vi "3Dmodel.vi"() -> (1 "SceneObject out":refnum<vi>, 2 "error out":errorcluster)   [LabVIEW 2021]
doc: "Creates the 3D scene with the lightsaber composed by two cylinders: the Blade and the Handle."
uses:
  <vilib>/picture/3D Picture Control/Object/Create Object (name).vi
  <vilib>/picture/3D Picture Control/NI_3D Picture Control.lvlib
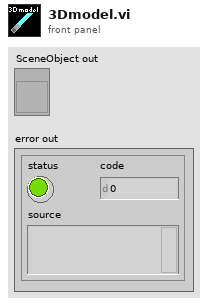
[diagram p1: front panel]
types:
  T1 = cluster{"Red":sgl, "Green":sgl, "Blue":sgl, "Alpha":sgl}
  T2 = enum16{"As a Decal", "With Modulation", "With Blending", "As a replacement"}
  T3 = typedef "imagedata.ctl" = cluster{"image type":i32, "image depth":i32, "image":u8[], "mask":u8[], "colors":u32[], "Rectangle":cluster{"left":i16, "top":i16, "right":i16, "bottom":i16}}
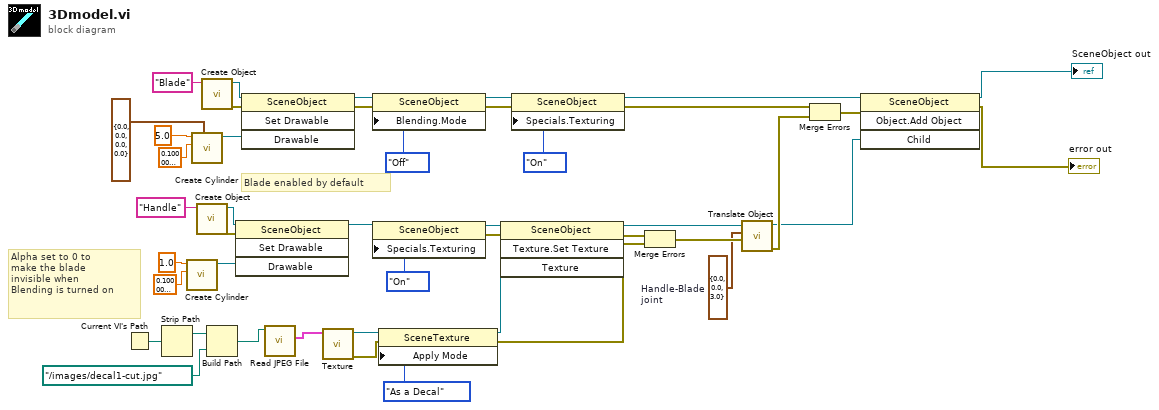
[diagram p0: block diagram]
diagram:
  w23 = cluster{"X":sgl, "Y":sgl, "Z":sgl} {"X"=0.0, "Y"=0.0, "Z"=3.0}  # Handle-Blade joint
  # "Blade enabled by default"
  # "Alpha set to 0 to \nmake the blade\ninvisible when \nBlending is turned on"
  n1 = Current VI's Path() -> (path=w5:path)
  n2 = Strip Path(path=w5) -> (stripped path=w6:path)  [unwired: 1 out]
  n3 = call <vilib>:"Create Cylinder.vi"("Radius"=sgl 0.1, "Height"=sgl 1.0) -> ("New Cylinder Refnum"=w22:refnum<vi>)  [unwired: 8 in, 1 out]
  n4 = call <vilib>:"Create Cylinder.vi"("Color"=T1 {"Red"=0.0, "Green"=0.0, "Blue"=0.0, "Alpha"=0.0}, "Radius"=sgl 0.1, "Height"=sgl 5.0) -> ("New Cylinder Refnum"=w19:refnum<vi>)  [unwired: 7 in, 1 out]
  n5 = call-poly <vilib>:"Create Object.vi"("Name"="Handle") -> ("error out"=w28:errorcluster, "Scene:New Object"=w25:refnum<vi>)  [unwired: 9 in]
  n6 = call-poly <vilib>:"Create Object.vi"("Name"="Blade") -> ("error out"=w14:errorcluster, "Scene:New Object"=w15:refnum<vi>)  [unwired: 9 in]
  n7 = Build Path(base path=w6, name or relative path=path "../images/decal1-cut.jpg" ("path to JPEG file")) -> (appended path=w3:path)
  n8 = invoke class="SceneObject" method="Set Drawable"(reference=w25, error in=w28, "Drawable"=w22) -> (reference out=w41:refnum<vi>)  [unwired: 1 in, 3 out]
  n9 = invoke class="SceneObject" method="Set Drawable"(reference=w15, error in=w14, "Drawable"=w19) -> (reference out=w13:refnum<vi>, error out=w12:errorcluster)  [unwired: 1 in, 2 out]
  n10 = call <vilib>:"Read JPEG File.vi"("path to JPEG file"=w3) -> ("image data"=w34:T3)  [unwired: 8 in, 2 out]
  n11 = call <vilib>:"Texture.vi"("Image"=w34) -> ("error out"=w36:errorcluster, "New Texture Refnum"=w35:refnum<vi>)  [unwired: 9 in]
  n12 = property on="Property Node" class="SceneObject"(reference=w13, error in=w12, "Blending.Mode"=enum16{"Inherit Value", "Off", "On"}."Off" ("Blending:Mode")) -> (reference out=w9:refnum<vi>, error out=w8:errorcluster)
  n13 = property class="SceneObject"(reference=w41, "Specials.Texturing"=enum16{"Inherit Value", "Off", "On"}."On" ("Specials:Texturing")) -> (reference out=w31:refnum<vi>, error out=w32:errorcluster)  [unwired: 1 in]
  n14 = property class="SceneTexture"(reference=w35, error in=w36, "Apply Mode"=T2."As a Decal") -> (reference out=w38:refnum<vi>, error out=w39:errorcluster)
  n15 = invoke class="SceneObject" method="Texture.Set Texture"(reference=w31, error in=w32, "Texture"=w38) -> (reference out=w42:refnum<vi>, error out=w40:errorcluster)  [unwired: 1 in, 2 out]
  n16 = property class="SceneObject"(reference=w9, error in=w8, "Specials.Texturing"=enum16{"Inherit Value", "Off", "On"}."On" ("Specials:Texturing")) -> (reference out=w2:refnum<vi>, error out=w1:errorcluster)
  n17 = Merge Errors(w40, w39) -> (w43:errorcluster)
  n18 = call <vilib>:"Translate Object.vi"("error in (no error)"=w43, "Translation"=w23, "Scene.Object In"=w42) -> ("error out"=w44:errorcluster, "Scene.Object Out"=w27:refnum<vi>)  [unwired: 7 in]
  n19 = Merge Errors(w1, w44) -> (w29:errorcluster)
  n20 = invoke class="SceneObject" method="Object.Add Object"(reference=w2, error in=w29, "Child"=w27) -> (reference out=→"SceneObject out":refnum<vi>, error out=→"error out":errorcluster)  [unwired: 1 in, 2 out]
